vi "Global_CMD Data.vi"() -> ()   [LabVIEW 2017, in "Overlords.lvlib"]
uses:
  Overlords.lvlib
  Cluster_CMD to SM Data.ctl
  ENUM_Overloard State.ctl
  <vilib>/Rock Robotics/WPI/DriverStation/WPI_DriverStationMatch Info.ctl
  Hopper/ENUM_Firing_State.ctl
  Hopper/Hopper System.lvlib
panel:
  in  "CMD_Overloard Data":T1={"Overloard State"=enum."Idle", "Match Info"={"Autonomous Elapsed Seconds"=0.0, "TeleOp Elapsed Seconds"=0.0, "Disabled Elapsed Seconds"=0.0, "Visited Autonomous"=FALSE, "Visited TeleOp"=FALSE, "Visited Disabled"=FALSE, "Autonomous Settings"={"Autonomous Style"=enum."Independent", "VI Refnum"=refnum}}, "Firing State"=enum."No Fireing", "Gear wait till pullback (seconds)"=0.0}
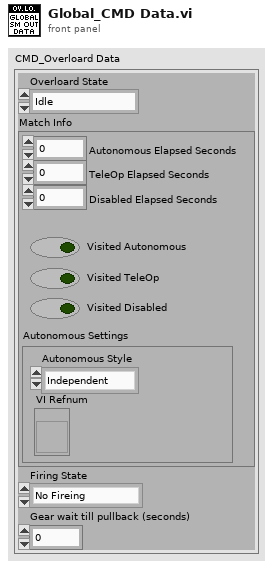
[diagram p1: front panel]
types:
  T1 = typedef "Overlords.lvlib/Cluster_CMD to SM Data.ctl" = cluster{"Overloard State":T2, "Match Info":T3, "Firing State":T4, "Gear wait till pullback (seconds)":dbl}
  T2 = typedef "Overlords.lvlib/ENUM_Overloard State.ctl" = enum16{"Idle", "High Shot", "Low Shot", "Place Gear", "Climb"}
  T3 = typedef "WPI_DriverStationMatch Info.ctl" = cluster{"Autonomous Elapsed Seconds":dbl, "TeleOp Elapsed Seconds":dbl, "Disabled Elapsed Seconds":dbl, "Visited Autonomous":bool, "Visited TeleOp":bool, "Visited Disabled":bool, "Autonomous Settings":cluster{"Autonomous Style":enum16{"Iterative", "Independent"}, "VI Refnum":refnum<vi>}}
  T4 = typedef "Hopper System.lvlib/ENUM_Firing_State.ctl" = enum16{"No Fireing", "Rapid Fire", "Shotgun Fireing"}
diagram:
